vi "Defeated Message.vi"(8 "error in (no error)":errorcluster, 11 "MyTeam in":refnum<class "MyTeam.lvclass">) -> (0 "error out":errorcluster, 2 "Defeated Message":string, 3 "MyTeam out":refnum<class "MyTeam.lvclass">)   [LabVIEW 2020, in "SquareTeam.lvlib" / "MyTeam.lvclass"]
uses:
  MyTeam.lvclass
  MyTeam.lvclass/MyTeam.ctl
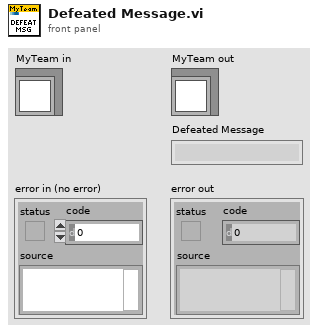
[diagram p1: front panel]
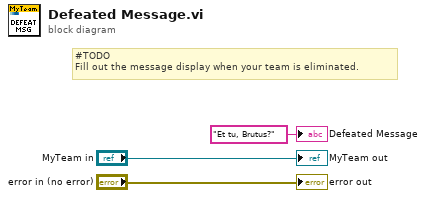
[diagram p0: block diagram]
diagram:
  # "#TODO\nFill out the message display when your team is eliminated."
  "error out" <- "error in (no error)"
  "MyTeam out" <- "MyTeam in"
  "Defeated Message" <- "Et tu, Brutus?" ("Defeated Message")
